vi "Actuator Volts Transaction List.vi"(5 "error in (no error)":errorcluster, 7 "Source":T1) -> (0 "error out":errorcluster, 3 "Transactions":string[](array[string]))   [LabVIEW 2013]
uses:
  Names/Source Group Type.ctl
panel:
  in  "Pattern":string="/Act/*"
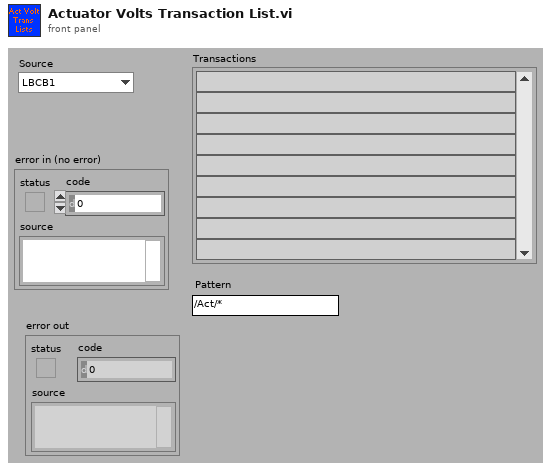
[diagram p1: front panel]
types:
  T1 = typedef "Source Group Type.ctl" = enum16{"LBCB1", "LBCB2", "Consolidated", "External"}
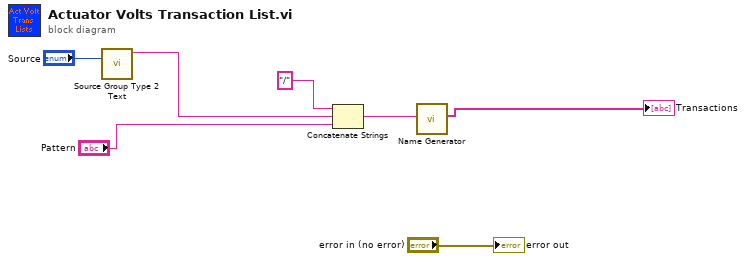
[diagram p0: block diagram]
diagram:
  n1 = call "Source Group Type 2 Text.vi"("Source"="Source") -> ("String"=w4:string)  [unwired: 10 in]
  n2 = Concatenate Strings("/" ("string"), w4, "Pattern") -> (w2:string)
  n3 = call "Name Generator.vi"("Group Specifier"=w2) -> ("Group Names"=→"Transactions":string[])  [unwired: 10 in]
  "error out" <- "error in (no error)"
